vi "Get Program revision.vi"() -> (3 "Revision":string)   [LabVIEW 2025]
uses:
  <vilib>/Utility/file.llb/Read Delimited Spreadsheet (string).vi
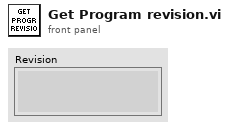
[diagram p1: front panel]
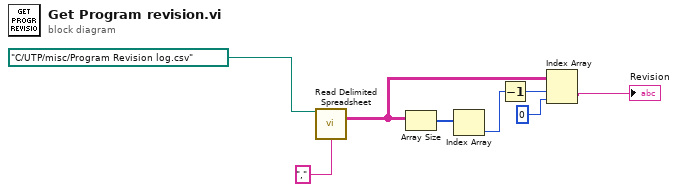
[diagram p0: block diagram]
diagram:
  n1 = call-poly <vilib>:"Read Delimited Spreadsheet.vi"("file path (dialog if empty)"=path "C:/UTP/misc/Program Revision log.csv", "delimiter (\\t)"="," ("delimiter (\\t)")) -> ("all rows"=w6:string[][])  [unwired: 8 in, 5 out]
  n2 = Array Size(array=w6) -> (size(s)=w5:i32[])
  n3 = Index Array(array=w5) -> (element=w4:i32)  [unwired: 1 in]
  n4 = Decrement(x=w4) -> (x-1=w3:i32)
  n5 = Index Array(array=w6, index (row)=w3, index (col)=0) -> (element=→"Revision":string)
